vi "Get Class.vi"(0 "listbox 输入":refnum<class "listbox.lvclass">, 2 "项标识符":string, 3 "error in (no error)":errorcluster caption="错误输入（无错误）") -> (7 "listbox 输出":refnum<class "listbox.lvclass">, 8 "Menu.lvclass":refnum<class "Menu.lvclass">, 10 "error out":errorcluster caption="错误输出")   [LabVIEW 2016, in "listbox.lvclass"]
uses:
  listbox.lvclass
  LNK/Parent Class/Menu.lvclass
  listbox.lvclass/listbox.ctl
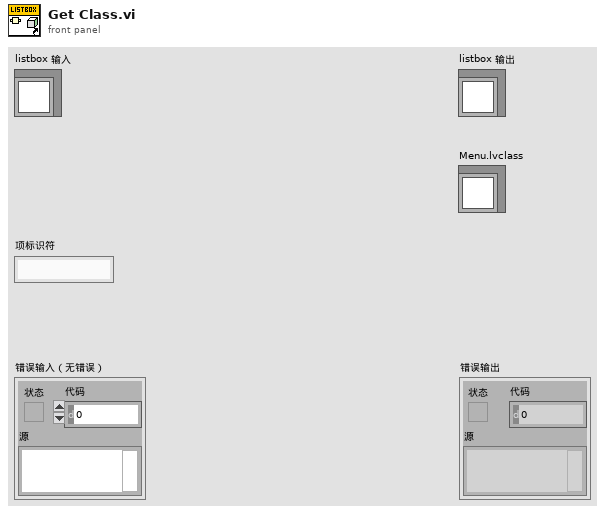
[diagram p1: front panel]
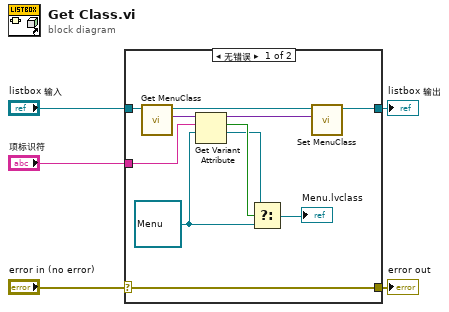
[diagram p0: block diagram]
diagram:
  n1 = case shown="无错误" "error in (no error)" {
    selector: "error in (no error)" -> [w15 w18]
    tunnel: [w15 w18] -> w4
    tunnel: [w13 w17] -> w2
    tunnel: "listbox 输入" -> [w16 w17]
    tunnel: "项标识符" -> [w6 _]
    frame No Error {
      w8 = refnum<class "Menu.lvclass"> refnum ("LNK.lvclass")
      n2 = call "Get MenuClass.vi"("listbox in"=w16) -> ("MenuClass"=w12:variant, "listbox out"=w14:refnum<class "listbox.lvclass">)  [unwired: 9 in]
      n3 = Get Variant Attribute(Variant=w12, name=w6, default value (empty Variant)=w8) -> (duplicate Variant=w11:variant, found=w10:bool, value=w9:refnum<class "Menu.lvclass">)  [unwired: 1 in, 1 out]
      n4 = Select(t=w9, s=w10, f=w8) -> (s? t:f=→"Menu.lvclass":refnum<class "Menu.lvclass">)
      n5 = call "Set MenuClass.vi"("MenuClass"=w11, "listbox in"=w14) -> ("listbox out"=w13:refnum<class "listbox.lvclass">)  [unwired: 9 in]
    }
    frame Error {
    }
  }
  "error out" <- w4
  "listbox 输出" <- w2
